vi "Conversion_into_SI_units.vi"(6 "Microsteps (MS=64)":dbl=64.0, 7 "Motor":u16(ring) items=["none", "1", "2", "3", "4", "all"], 8 "Input Unit":T1=enum."Meter", 10 "Input":dbl) -> (2 "Output":dbl)   [LabVIEW 2013]
uses:
  ConversionAndInformation/Unit_Control.ctl
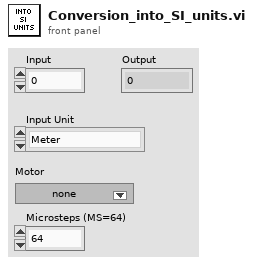
[diagram p1: front panel]
types:
  T1 = typedef "Unit_Control.ctl" = enum16{"Angle (Degrees)", "Rad", "Angle [TMC]", "Microsteps [TMC]", "Inches", "Nanometer", "Meter", "Centimeter", "Millimeter", "Micron", "Joule", "Electron Volts", "Hertz", "Terahertz", "Megahertz"}
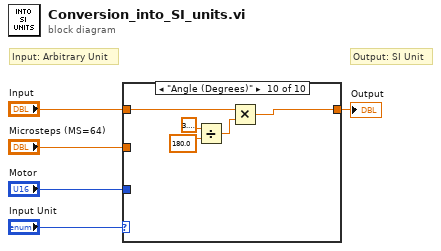
[diagram p0: block diagram]
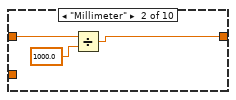
[diagram p3: hidden frame]
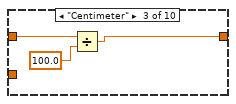
[diagram p4: hidden frame]
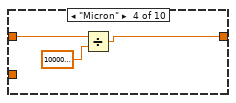
[diagram p5: hidden frame]
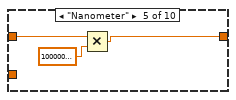
[diagram p6: hidden frame]
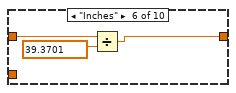
[diagram p7: hidden frame]
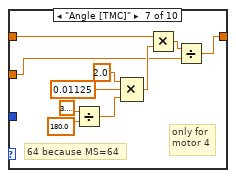
[diagram p8: hidden frame]
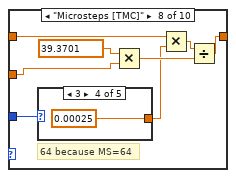
[diagram p9: hidden frame]
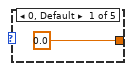
[diagram p10: hidden frame]
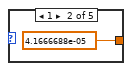
[diagram p11: hidden frame]
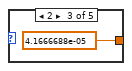
[diagram p12: hidden frame]
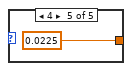
[diagram p13: hidden frame]
diagram:
  # "Output: SI Unit"
  # "Input: Arbitrary Unit"
  n1 = case shown="\"Angle (Degrees)\"" "Input Unit" {
    tunnel: "Input" -> [w6 w9 w12 w15 w18 w20 w30 w36 w45 w48]
    tunnel: [w6 w8 w10 w14 w16 w19 w29 w35 w45 w46] -> w5
    tunnel: "Motor" -> [_ _ _ _ _ _ _ w34 _ _]
    tunnel: "Microsteps (MS=64)" -> [_ _ _ _ _ _ w22 w33 _ _]
    frame "Meter", Default {
    }
    frame "Millimeter" {
      n2 = Divide(x=w9, y=1000.0) -> (x/y=w8:dbl)
    }
    frame "Centimeter" {
      n3 = Divide(x=w12, y=100.0) -> (x/y=w10:dbl)
    }
    frame "Micron" {
      n4 = Divide(x=w15, y=1000000.0) -> (x/y=w14:dbl)
    }
    frame "Nanometer" {
      n5 = Multiply(x=w18, y=1000000000000.0) -> (x*y=w16:dbl)
    }
    frame "Inches" {
      n6 = Divide(x=w20, y=39.3701) -> (x/y=w19:dbl)
    }
    frame "Angle [TMC]" {
      # "only for\nmotor 4"
      # "64 because MS=64"
      n7 = Divide(x=3.141592653589793, y=180.0) -> (x/y=w24:dbl)
      n8 = Compound Arithmetic op=MULTIPLY(2.0 ("x"), 0.01125, w24) -> (w23:dbl)
      n9 = Multiply(x=w30, y=w23) -> (x*y=w31:dbl)
      n10 = Divide(x=w31, y=w22) -> (x/y=w29:dbl)
    }
    frame "Microsteps [TMC]" {
      # "64 because MS=64"
      n11 = case shown="3" w34 {
        tunnel: [0.0 4.1666688e-05 4.1666688e-05 0.00025 0.0225] -> w32
        frame 0, Default {
        }
        frame 1 {
        }
        frame 2 {
        }
        frame 3 {
        }
        frame 4 {
        }
      }
      n12 = Multiply(x=39.3701, y=w33) -> (x*y=w37:dbl)
      n13 = Multiply(x=w36, y=w32) -> (x*y=w39:dbl)
      n14 = Divide(x=w39, y=w37) -> (x/y=w35:dbl)
    }
    frame "Rad" {
    }
    frame "Angle (Degrees)" {
      n15 = Divide(x=3.141592653589793, y=180.0) -> (x/y=w47:dbl)
      n16 = Multiply(x=w48, y=w47) -> (x*y=w46:dbl)
    }
  }
  "Output" <- w5
